vi "RH_DCPower_Measure.vi"(8 "error in (no error)":errorcluster, 10 "channel name":string, 11 "DCPower Session In":refnum<k15>) -> (0 "error out":errorcluster, 1 "Current":dbl, 2 "Voltage":dbl, 3 "DCPower Session Out":refnum<k15>)   [LabVIEW 2023, in "ResourceHandling.lvlib"]
doc: "Measures On Demand Voltage and Current"
uses:
  ResourceHandling.lvlib
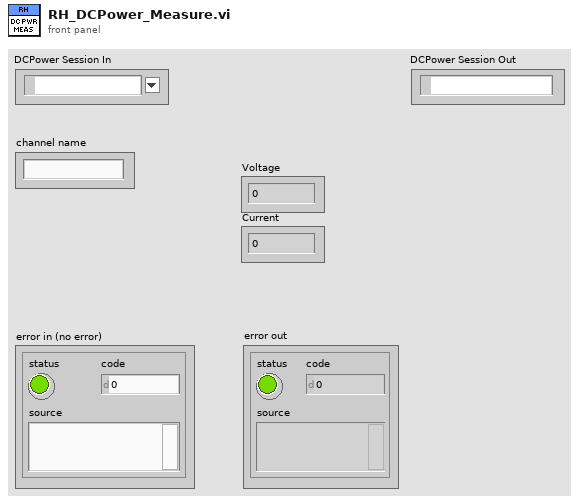
[diagram p1: front panel]
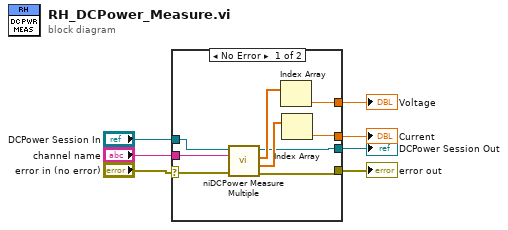
[diagram p0: block diagram]
diagram:
  n1 = case shown="No Error" "error in (no error)" {
    selector: "error in (no error)" -> [w14 w17]
    tunnel: [w12 w17] -> w7
    tunnel: [w11 w18] -> w2
    tunnel: "DCPower Session In" -> [w13 w18]
    tunnel: [w10 _] -> w5
    tunnel: [w9 _] -> w4
    tunnel: "channel name" -> [w8 _]
    frame No Error {
      n2 = call <instrlib>:"niDCPower Measure Multiple.vi"("error in (no error)"=w14, "channel name"=w8, "instrument handle"=w13) -> ("error out"=w12:errorcluster, "current measurements"=w16:dbl[], "voltage measurements"=w15:dbl[], "instrument handle out"=w11:refnum<k15>)  [unwired: 5 in]
      n3 = Index Array(array=w15) -> (element=w10:dbl)  [unwired: 1 in]
      n4 = Index Array(array=w16) -> (element=w9:dbl)  [unwired: 1 in]
    }
    frame Error {
    }
  }
  "error out" <- w7
  "Voltage" <- w5
  "Current" <- w4
  "DCPower Session Out" <- w2
